vi "Test Passing.vi"(8 "error in (no error)":errorcluster, 11 "Passing Test Case In":refnum<class "Passing Test Case.lvclass">) -> (0 "error out":errorcluster, 3 "Passing Test Case Out":refnum<class "Passing Test Case.lvclass">)   [LabVIEW 2020, in "Passing Test Case.lvclass"]
doc: "Passing test"
uses:
  Passing Test Case.lvclass
  LUnit Test Case.lvclass
  C:/git/astemes-lunit/source/LUnit Test Case.lvclass
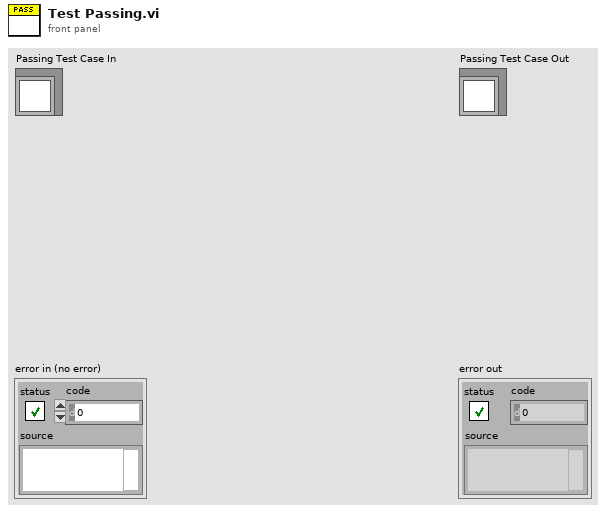
[diagram p1: front panel]
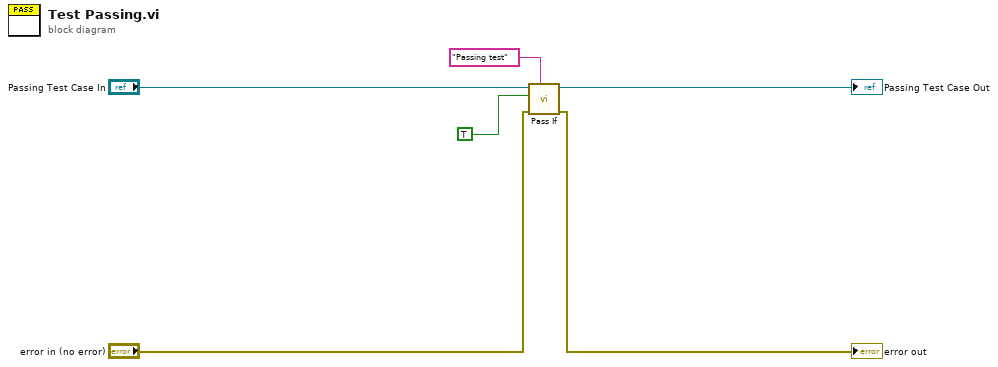
[diagram p0: block diagram]
diagram:
  n1 = call "Pass If.vi"("Description"="Passing test", "error in (no error)"="error in (no error)", "Pass?"=TRUE, "LUnit Test Case In"="Passing Test Case In") -> ("error out"=→"error out":errorcluster, "LUnit Test Case Out"=→"Passing Test Case Out":refnum<class "Passing Test Case.lvclass">)  [unwired: 6 in]
